vi "HH_CalcTimeTrace.vi"(4 "Channel":i32, 5 "Bin":i32, 6 "ChannelsZero":u32[](array[numeric]), 7 "LengthTTrace":u64, 9 "NumChannels":i32, 10 "TimeTraces in":u32[][](array[numeric]), 11 "DeltaTotalBin":u64) -> (3 "TimeTraces out":u32[][](array[numeric]))   [LabVIEW 2017]
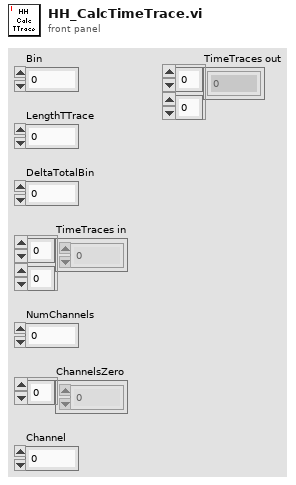
[diagram p1: front panel]
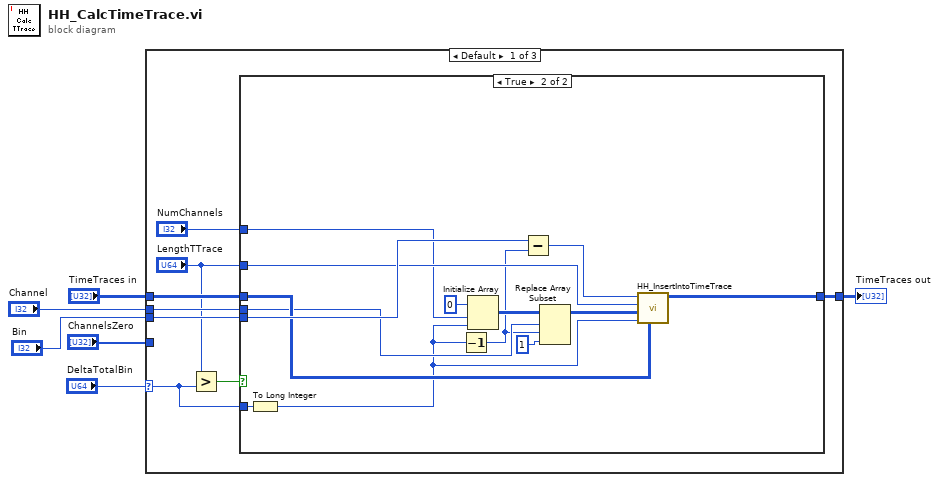
[diagram p0: block diagram]
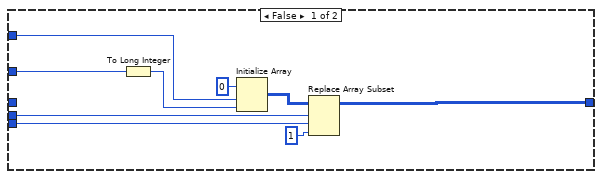
[diagram p2: hidden frame]
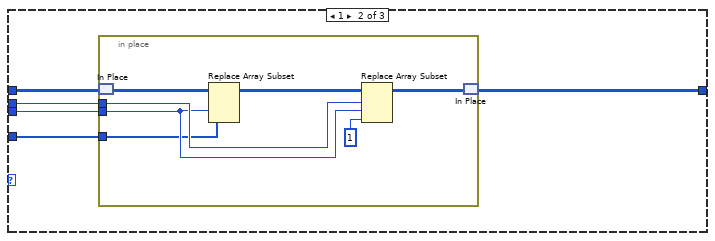
[diagram p3: hidden frame]
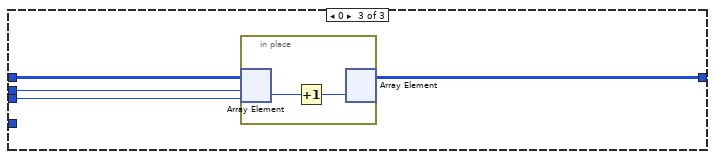
[diagram p4: hidden frame]
diagram:
  n1 = case shown="Default" "DeltaTotalBin" {
    selector: "DeltaTotalBin" -> [w10 _ _]
    tunnel: "Bin" -> [w13 w41 w51]
    tunnel: [w14 w38 w53] -> w3
    tunnel: "TimeTraces in" -> [w12 w39 w52]
    tunnel: "Channel" -> [w11 w42 w50]
    tunnel: "ChannelsZero" -> [_ w40 _]
    frame Default {
      n2 = Greater?(x="LengthTTrace", y=w10) -> (0:w9:bool)
      n3 = case shown="True" w9 {
        tunnel: [w23 w35] -> w14
        tunnel: w10 -> [_ w37]
        tunnel: w13 -> [w21 w36]
        tunnel: "LengthTTrace" -> [w22 w34]
        tunnel: w11 -> [w20 w31]
        tunnel: w12 -> [_ w33]
        tunnel: "NumChannels" -> [w19 w32]
        frame False {
          n4 = To Long Integer(number=w22) -> (32bit integer=w15:i32)
          n5 = Initialize Array(u32 0 ("element"), w19, w15) -> (w17:u32[][])
          n6 = Replace Array Subset(array=w17, new element=u32 1 ("new element/subarray"), index (row)=w20, index (col)=w21) -> (w23:u32[][])
        }
        frame True {
          n7 = To Long Integer(number=w37) -> (32bit integer=w28:i32)
          n8 = Decrement(x=w28) -> (x-1=w26:i32)
          n9 = Initialize Array(u32 0 ("element"), w32, w28) -> (w27:u32[][])
          n10 = Subtract(x=w36, y=w26) -> (x-y=w29:i32)
          n11 = Replace Array Subset(array=w27, new element=u32 1, index (row)=w31, index (col)=w26) -> (w24:u32[][])
          n12 = call "HH_InsertIntoTimeTrace.vi"("TimeTrace in"=w33, "NumVals"=w28, "Vals"=w24, "LengthTTrace"=w34, "TimeTraceBin"=w29) -> ("TimeTrace out"=w35:u32[][])  [unwired: 6 in]
        }
      }
    }
    frame 1 {
      n13 = in-place {
        in-place-border: w42 -> [w47]
        in-place-border: w41 -> [w46]
        in-place-border: w40 -> [w45]
        n14 = in-place-match #1(w39) -> (w44:u32[][])
        n15 = Replace Array Subset(array=w44, new element=w45, index (col)=w46) -> (w49:u32[][])  [unwired: 1 in]
        n16 = Replace Array Subset(array=w49, new element=u32 1 ("new element/subarray"), index (row)=w47, index (col)=w46) -> (w43:u32[][])
        n17 = in-place-match #1(w43) -> (w38:u32[][])
      }
    }
    frame 0 {
      n18 = in-place {
        n19 = in-place-array #2(w52, w50, w51) -> (w55:u32)
        n20 = Increment(x=w55) -> (x+1=w54:u32)
        n21 = in-place-array #2(w54) -> (w53:u32[][])  [unwired: 2 out]
      }
    }
  }
  "TimeTraces out" <- w3
